vi "Vision System.vi"() -> ()   [LabVIEW 2017]
uses:
  <vilib>/userdefined/High Color/IMAQdx.ctl
  <vilib>/vision/driver/NI_Vision_Acquisition_Software.lvlib
panel:
  out "error out 3":errorcluster
  out "error out 2":errorcluster
  out "Image":T1(plugin-control)
  out "error out":errorcluster
  in  "Session In":T2
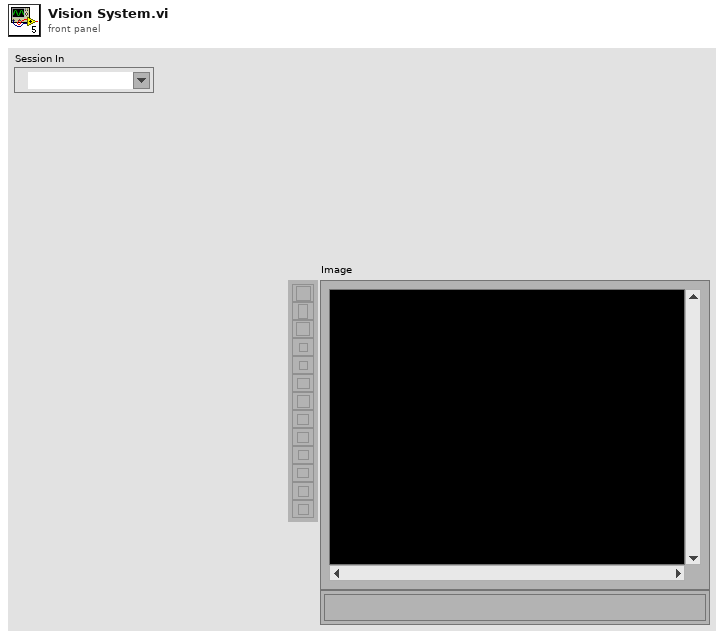
[diagram p1: front panel]
types:
  T1 = typedef "IMAQ Image.ctl" = refnum<image>
  T2 = typedef "IMAQdx.ctl" = refnum<k21>
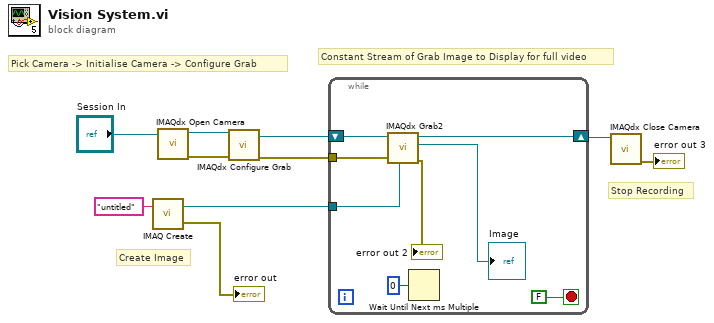
[diagram p0: block diagram]
diagram:
  # "Create Image"
  # "Stop Recording"
  # "Constant Stream of Grab Image to Display for full video"
  # "Pick Camera -> Initialise Camera -> Configure Grab"
  n1 = call "IMAQ Create"("Image Name"="untitled") -> ("New Image"=w7:T1, "error out"=→"error out":errorcluster)  [unwired: 4 in]
  n2 = call <vilib>:"IMAQdx Open Camera.vi"("Session In"="Session In") -> ("error out"=w9:errorcluster, "Session Out"=w10:T2)  [unwired: 9 in]
  n3 = call <vilib>:"IMAQdx Configure Grab.vi"("error in"=w9, "Session In"=w10) -> ("error out"=w3:errorcluster, "Session Out"=w8:T2)  [unwired: 8 in]
  n4 = while {
    tunnel: w7 -> [w17]
    shift-right: [w15] -> w4
    shift-left: w8 -> [w18]
    tunnel: w3 -> [w13]
    stop <- FALSE stop-if-true
    n5 = call <vilib>:"IMAQdx Grab2.vi"("error in"=w13, "Image In"=w17, "Session In"=w18) -> ("error out"=→"error out 2":errorcluster, "Image Out"=→"Image":T1, "Session Out"=w15:T2)  [unwired: 5 in, 1 out]
    n6 = Wait Until Next ms Multiple(millisecond multiple=u32 0) -> ()  [unwired: 1 out]
  }
  n7 = call <vilib>:"IMAQdx Close Camera.vi"("Session In"=w4) -> ("error out"=→"error out 3":errorcluster)  [unwired: 10 in]
